vi "Activity Log.vi"(6 "Log File Path":path, 7 "Action":T1, 8 "Error In":errorcluster, 9 "string ref":refnum<vi>, 11 "Message Log Entry":string) -> (0 "Error Out":errorcluster, 3 "Message Log":string)   [LabVIEW 2021]
doc: "This functional global timestamps and records text messages for a generic message log."
uses:
  Activity Log enum Action .ctl
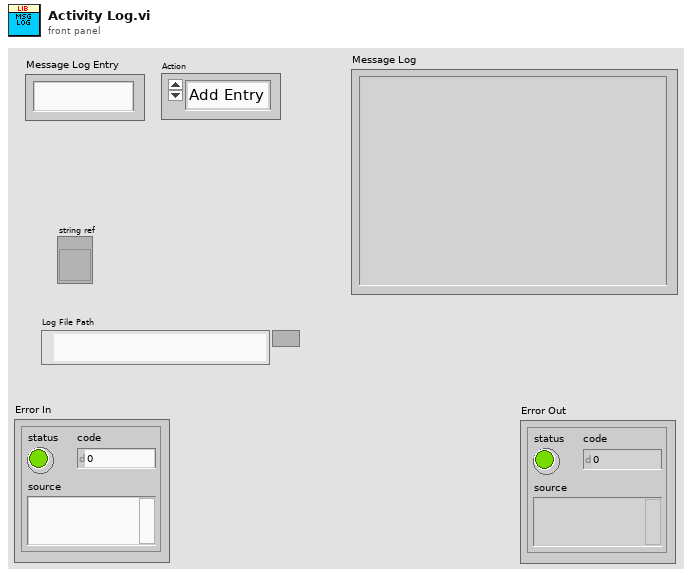
[diagram p1: front panel]
types:
  T1 = typedef "Activity Log enum Action .ctl" = enum16{"Add Entry", "Get Log", "Restore From Disk", "Save to Disk", "Init"}
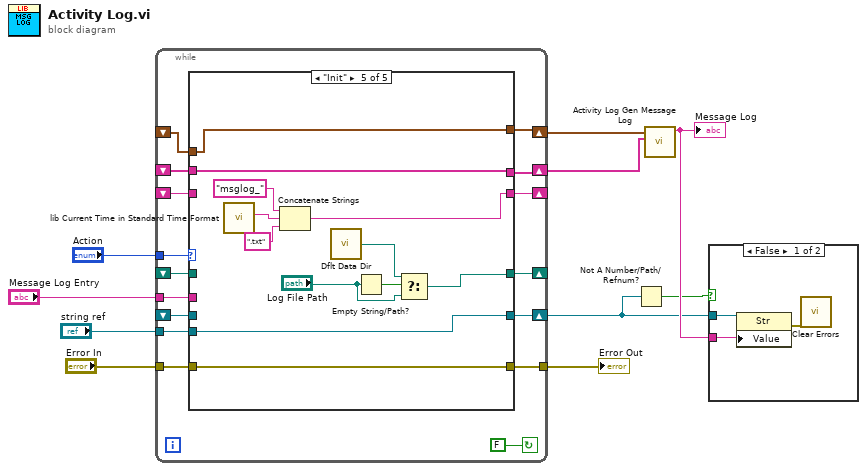
[diagram p0: block diagram]
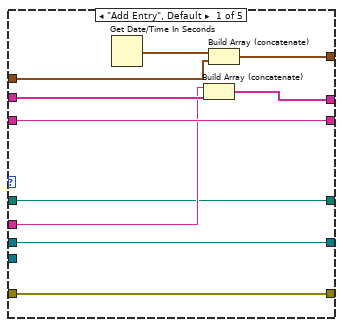
[diagram p3: hidden frame]
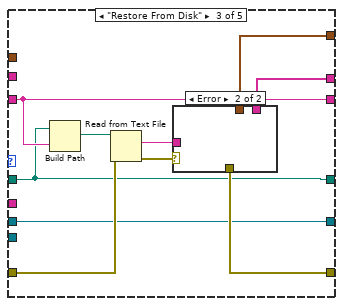
[diagram p5: hidden frame]
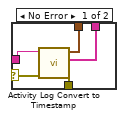
[diagram p6: hidden frame]
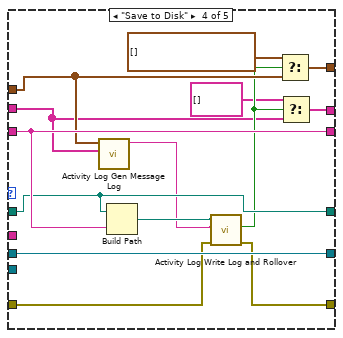
[diagram p7: hidden frame]
diagram:
  n1 = while {
    tunnel: "Action" -> [w26]
    shift-right: [w22] -> w6
    shift-left: _ -> [w21]
    shift-right: [w23] -> w5
    shift-left: _ -> [w20]
    tunnel: "Message Log Entry" -> [w24]
    tunnel: "Error In" -> [w19]
    tunnel: [w18] -> w7
    shift-right: [w17] -> _
    shift-left: _ -> [w16]
    shift-right: [w15] -> w2
    shift-left: _ -> [w13]
    tunnel: "string ref" -> [w14]
    shift-right: [w12] -> _
    shift-left: _ -> [w11]
    stop <- FALSE continue-if-true
    n2 = case shown="\"Init\"" w26 {
      tunnel: w24 -> [w30 _ _ _ _]
      tunnel: [w36 w42 w47 w59 w81] -> w23
      tunnel: [w35 w41 w48 w62 w83] -> w22
      tunnel: w21 -> [w29 w41 _ w64 w83]
      tunnel: w20 -> [w34 w42 _ w60 w81]
      tunnel: w19 -> [w33 w40 w50 w68 w82]
      tunnel: [w33 w40 w49 w67 w82] -> w18
      tunnel: [w32 w39 w46 w71 w72] -> w17
      tunnel: w16 -> [w32 w39 w46 w71 _]
      tunnel: [w31 w38 w45 w70 w80] -> w15
      tunnel: w14 -> [_ _ _ _ w80]
      tunnel: w13 -> [w31 w38 w45 w70 _]
      tunnel: [w27 w37 w44 w69 w76] -> w12
      tunnel: w11 -> [w27 w37 w44 w69 _]
      frame "Add Entry", Default {
        n3 = Get Date/Time In Seconds() -> (seconds since 1Jan1904=w28:timestamp)
        n4 = Build Array (concatenate)(w30, w34) -> (w36:string[])
        n5 = Build Array (concatenate)(w28, w29) -> (w35:timestamp[])
      }
      frame "Get Log" {
      }
      frame "Restore From Disk" {
        n6 = Build Path(base path=w44, name or relative path=w46) -> (appended path=w52:path)
        n7 = Read from Text File(file (use dialog)=w52, error in=w50) -> (text=w51:string, error out=w43:errorcluster)  [unwired: 2 in, 2 out]
        n8 = case shown="Error" w43 {
          selector: w43 -> [w53 _]
          tunnel: w51 -> [w57 _]
          tunnel: [w56 _] -> w49
          tunnel: [w55 _] -> w48
          tunnel: [w54 _] -> w47
          frame No Error {
            n9 = call "Activity Log Convert to Timestamp.vi"("error in (no error)"=w53, "Message Log"=w57) -> ("error out"=w56:errorcluster, "Messages"=w54:string[], "timestamps"=w55:timestamp[])  [unwired: 7 in]
          }
          frame Error {
          }
        }
      }
      frame "Save to Disk" {
        n10 = call "Activity Log Gen Message Log.vi"("Messages"=w60, "Timestamps"=w64) -> ("Message Log"=w65:string)  [unwired: 8 in, 1 out]
        n11 = Build Path(base path=w69, name or relative path=w71) -> (appended path=w66:path)
        n12 = call "Activity Log Write Log and Rollover.vi"("error in (no error)"=w68, "Log Text"=w65, "Log File"=w66) -> ("error out"=w67:errorcluster, "new file?"=w61:bool)  [unwired: 6 in, 1 out]
        n13 = Select(t=timestamp[] [], s=w61, f=w64) -> (s? t:f=w62:timestamp[])
        n14 = Select(t=string[] [], s=w61, f=w60) -> (s? t:f=w59:string[])
      }
      frame "Init" {
        n15 = call "lib Current Time in Standard Time Format.vi"() -> ("date/time string"=w75:string)  [unwired: 11 in]
        n16 = Concatenate Strings("msglog_" ("string"), w75, ".txt" ("string")) -> (w72:string)
        n17 = call <vilib>:"Dflt Data Dir.vi"() -> ("App:Default Data Directory"=w77:path)
        n18 = Empty String/Path?(string/path="Log File Path") -> (empty?=w79:bool)
        n19 = Select(t=w77, s=w79, f="Log File Path") -> (s? t:f=w76:path)
      }
    }
  }
  "Error Out" <- w7
  n20 = Not A Number/Path/Refnum?(number/path/refnum=w2) -> (NaN/Path/Refnum?=w1:bool)
  n21 = call "Activity Log Gen Message Log.vi"("Messages"=w5, "Timestamps"=w6) -> ("Message Log"=w3:string)  [unwired: 8 in, 1 out]
  "Message Log" <- w3
  n22 = case shown="False" w1 {
    tunnel: w3 -> [w86 _]
    tunnel: w2 -> [w85 _]
    frame False {
      n23 = property class="Str"(reference=w85, "Value"=w86) -> (error out=w84:errorcluster)  [unwired: 1 in, 1 out]
      n24 = call <vilib>:"Clear Errors.vi"("error in (no error)"=w84) -> ()  [unwired: 5 in, 2 out]
    }
    frame True {
    }
  }
